vi "Initialize Score Matrix.vi"(11 "Data Matrix":u8[][](array[numeric])) -> (1 "Columns":i32, 2 "Rows":i32, 3 "Score Matrix":u32[][](array[numeric]))   [LabVIEW 2019, in "Day 15.lvlib"]
uses:
  Day 15.lvlib
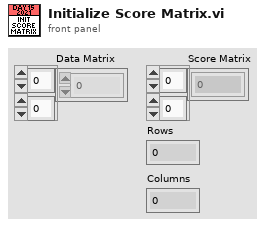
[diagram p1: front panel]
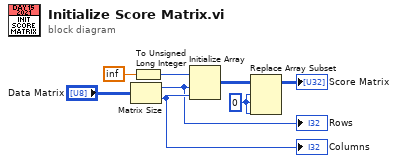
[diagram p0: block diagram]
diagram:
  w4 = 0 ("disabled index (col)")
  n1 = Matrix Size(0:"Data Matrix") -> (1:w7:i32, 2:w8:i32)
  "Columns" <- w8
  "Rows" <- w7
  n2 = To Unsigned Long Integer(number=inf) -> (unsigned 32bit integer=w2:u32)
  n3 = Initialize Array(w2, w7, w8) -> (w3:u32[][])
  n4 = Replace Array Subset(array=w3, new element=w4, index (row)=w4, index (col)=w4) -> (→"Score Matrix":u32[][])
